vi "schedule_triggers.vi"(8 "error in (no error)":errorcluster, 10 "new schedule entries":T1[](array[typedef]), 11 "DL090130ExperimentController in":refnum<class "ExperimentControllerDL090130Interval.lvclass">) -> (0 "error out":errorcluster, 3 "DL090130ExperimentController out":refnum<class "ExperimentControllerDL090130Interval.lvclass">)   [LabVIEW 2010, in "ExperimentControllerDL090130Interval.lvclass"]
uses:
  ExperimentControllerDL090130Interval.lvclass
  schedule_entry_cluster.ctl
  internal_trigger_enum.ctl
  ExperimentControllerDL090130Interval.lvclass/ExperimentControllerDL090130Interval.ctl
  common/classes/ErrorController/ErrorController/class_data.vi
  common/classes/ErrorController/ErrorController/ErrorController.lvclass
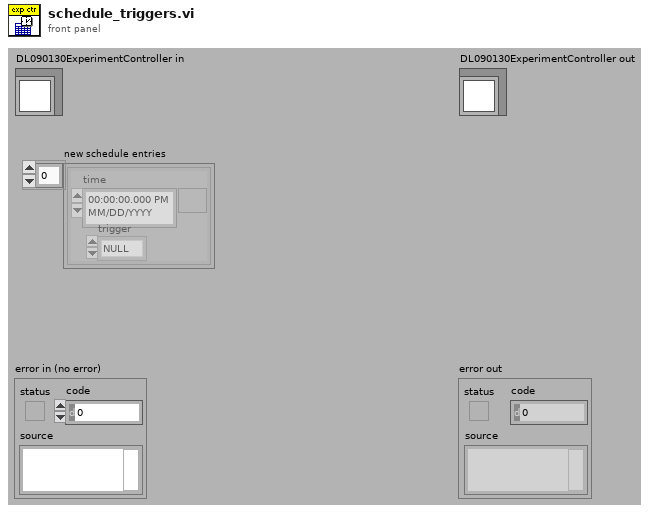
[diagram p1: front panel]
types:
  T1 = typedef "ExperimentControllerDL090130Interval.lvclass/schedule_entry_cluster.ctl" = cluster{"time":timestamp, "trigger":T2}
  T2 = typedef "ExperimentControllerDL090130Interval.lvclass/internal_trigger_enum.ctl" = enum16{"NULL", "initialise", "terminate", "start", "stop", "proceed", "prepare", "start sweep"}
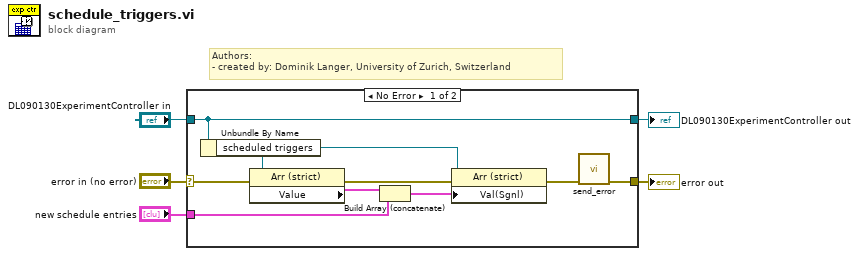
[diagram p0: block diagram]
diagram:
  # "Authors: \n- created by: Dominik Langer, University of Zurich, Switzerland"
  n1 = case shown="No Error" "error in (no error)" {
    selector: "error in (no error)" -> [w9 w16]
    tunnel: [w6 w16] -> w4
    tunnel: [w10 w15] -> w2
    tunnel: "DL090130ExperimentController in" -> [w10 w15]
    tunnel: "new schedule entries" -> [w8 _]
    frame No Error {
      n2 = Unbundle By Name(w10) -> ("scheduled triggers"=w12:refnum<vi>)
      n3 = property class="Arr (strict)"(reference=w12, error in=w9) -> (error out=w13:errorcluster, "Value"=w11:T1[])  [unwired: 1 out]
      n4 = Build Array (concatenate)(w11, w8) -> (w14:T1[])
      n5 = property class="Arr (strict)"(reference=w12, error in=w13, "Val(Sgnl)"=w14) -> (error out=w7:errorcluster)  [unwired: 1 out]
      n6 = call "send_error.vi"("error in (no error)"=w7) -> ("error out"=w6:errorcluster)  [unwired: 10 in]
    }
    frame Error {
    }
  }
  "error out" <- w4
  "DL090130ExperimentController out" <- w2
